vi "licznik.vi"(1 "kolumny":i32, 2 "wiersze":i32, 3 "Array":i32[][](array[numeric])) -> (0 "licznik":i32)   [LabVIEW 2016]
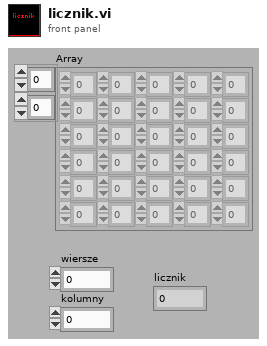
[diagram p1: front panel]
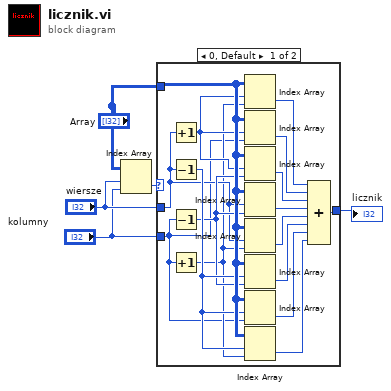
[diagram p0: block diagram]
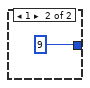
[diagram p2: hidden frame]
diagram:
  n1 = Index Array(array="Array", index (row)="wiersze", index (col)="kolumny") -> (element=w5:i32)
  n2 = case shown="0, Default" w5 {
    tunnel: "Array" -> [w21 _]
    tunnel: "wiersze" -> [w9 _]
    tunnel: "kolumny" -> [w7 _]
    tunnel: [w6 9] -> w1
    frame 0, Default {
      n3 = Increment(x=w9) -> (x+1=w10:i32)
      n4 = Decrement(x=w9) -> (x-1=w20:i32)
      n5 = Decrement(x=w7) -> (x-1=w19:i32)
      n6 = Increment(x=w7) -> (x+1=w8:i32)
      n7 = Index Array(array=w21, index (row)=w10, index (col)=w8) -> (element=w18:i32)
      n8 = Index Array(array=w21, index (row)=w10, index (col)=w7) -> (element=w17:i32)
      n9 = Index Array(array=w21, index (row)=w10, index (col)=w19) -> (element=w16:i32)
      n10 = Index Array(array=w21, index (row)=w9, index (col)=w19) -> (element=w15:i32)
      n11 = Index Array(array=w21, index (row)=w9, index (col)=w8) -> (element=w11:i32)
      n12 = Index Array(array=w21, index (row)=w20, index (col)=w19) -> (element=w12:i32)
      n13 = Index Array(array=w21, index (row)=w20, index (col)=w7) -> (element=w13:i32)
      n14 = Index Array(array=w21, index (row)=w20, index (col)=w8) -> (element=w14:i32)
      n15 = Compound Arithmetic op=ADD(w18, w17, w16, w15, w11, w12, w13, w14) -> (w6:i32)
    }
    frame 1 {
    }
  }
  "licznik" <- w1
